vi "xps_panel_destroy_ui_events.vi"(8 "error in (no error)":errorcluster, 11 "newport_xps_panel in":refnum<class "newport_xps_panel.lvclass">) -> (0 "error out":errorcluster, 3 "newport_xps_panel out":refnum<class "newport_xps_panel.lvclass">)   [LabVIEW 2015, in "newport_xps_panel.lvclass"]
uses:
  newport_xps_panel.lvclass
  newport_xps_panel.lvclass/newport_xps_panel.ctl
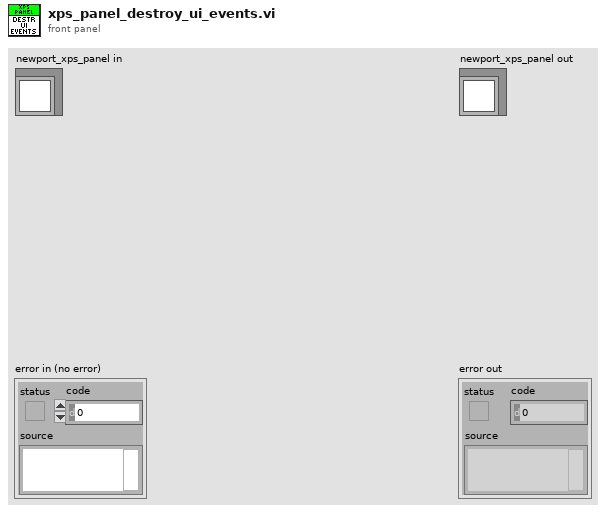
[diagram p1: front panel]
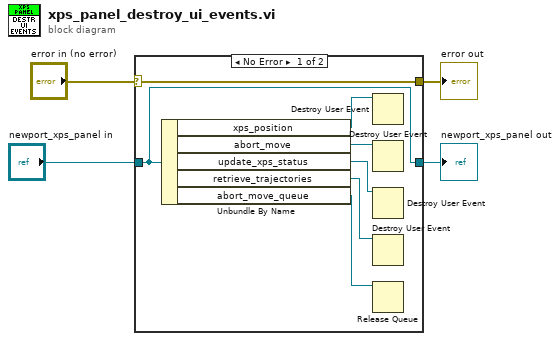
[diagram p0: block diagram]
diagram:
  n1 = case shown="No Error" "error in (no error)" {
    selector: "error in (no error)" -> [w11 w13]
    tunnel: [w11 w13] -> w3
    tunnel: [w10 w12] -> w1
    tunnel: "newport_xps_panel in" -> [w10 w12]
    frame No Error {
      n2 = Unbundle By Name(w10) -> ("xps_position"=w9:refnum<user-event>, "abort_move"=w8:refnum<user-event>, "update_xps_status"=w7:refnum<user-event>, "retrieve_trajectories"=w6:refnum<user-event>, "abort_move_queue"=w5:refnum<queue>)
      n3 = Destroy User Event(user event=w9) -> ()  [unwired: 1 in, 1 out]
      n4 = Destroy User Event(user event=w8) -> ()  [unwired: 1 in, 1 out]
      n5 = Destroy User Event(user event=w7) -> ()  [unwired: 1 in, 1 out]
      n6 = Destroy User Event(user event=w6) -> ()  [unwired: 1 in, 1 out]
      n7 = Release Queue(queue=w5) -> ()  [unwired: 2 in, 3 out]
    }
    frame Error {
    }
  }
  "error out" <- w3
  "newport_xps_panel out" <- w1
